vi "final-joystick.vi"() -> ()   [LabVIEW 2017]
uses:
  <vilib>/DAQmx/read.llb/DAQmx Read (Analog DBL 1Chan 1Samp).vi
  <vilib>/Utility/file.llb/Write Delimited Spreadsheet (string).vi
  <vilib>/Utility/file.llb/Read Delimited Spreadsheet (string).vi
  <vilib>/Utility/NIReport.llb/Append Report Text (str wrap).vi
  <vilib>/Utility/NIReport.llb/Append Text Table to Report (wrap).vi
  <vilib>/Utility/NIReport.llb/Append Image to Report (path wrap).vi
  <vilib>/DAQmx/create/channels.llb/DAQmx Create Channel (AI-Voltage-Basic).vi
  <vilib>/DAQmx/miscellaneous.llb/DAQmx Fill In Error Info.vi
  <vilib>/Utility/NIReport.llb/NI_report.lvclass
panel:
  in  "pos":string
  in  "x/y":string
  in  "File Path":path
  out "Array":string[][](array[string])
  out "Voltage Value":dbl(graph)
  out "Stop\nindicator":bool
  in  "LOG":bool
  out "Output Voltage":dbl format="%0.2f"
  in  "Stop Acquisition":bool
  in  "Input Channel":tag
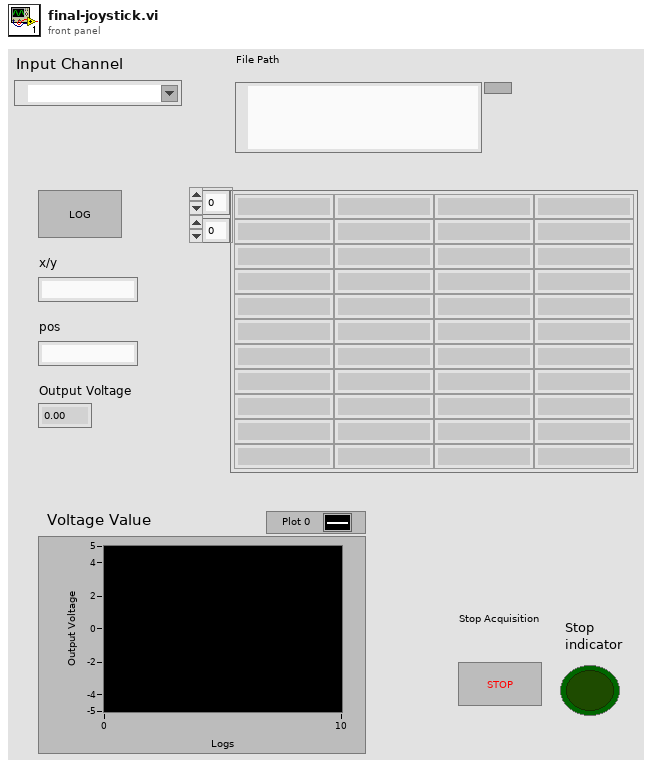
[diagram p1: front panel]
types:
  T1 = cluster{"Italic":enum16{"Italic Unchanged", "Italic On", "Italic Off"}, "Strike Through":enum16{"Strike Through Unchanged", "Strike Through On", "Strike Through Off"}, "Underline":enum16{"Underline Unchanged", "Underline On", "Underline Off"}, "Bold":enum16{"Bold Unchanged", "Bold On", "Bold Off"}}
  T2 = cluster{"Charset (-1)":i16, "Weight (-1)":i16, "Name":string, "Size":string}
  T3 = enum16{"maximized", "minimized", "normal", "no change"}
  T4 = enum16{"Standard Report", "HTML", "Word", "Excel"}
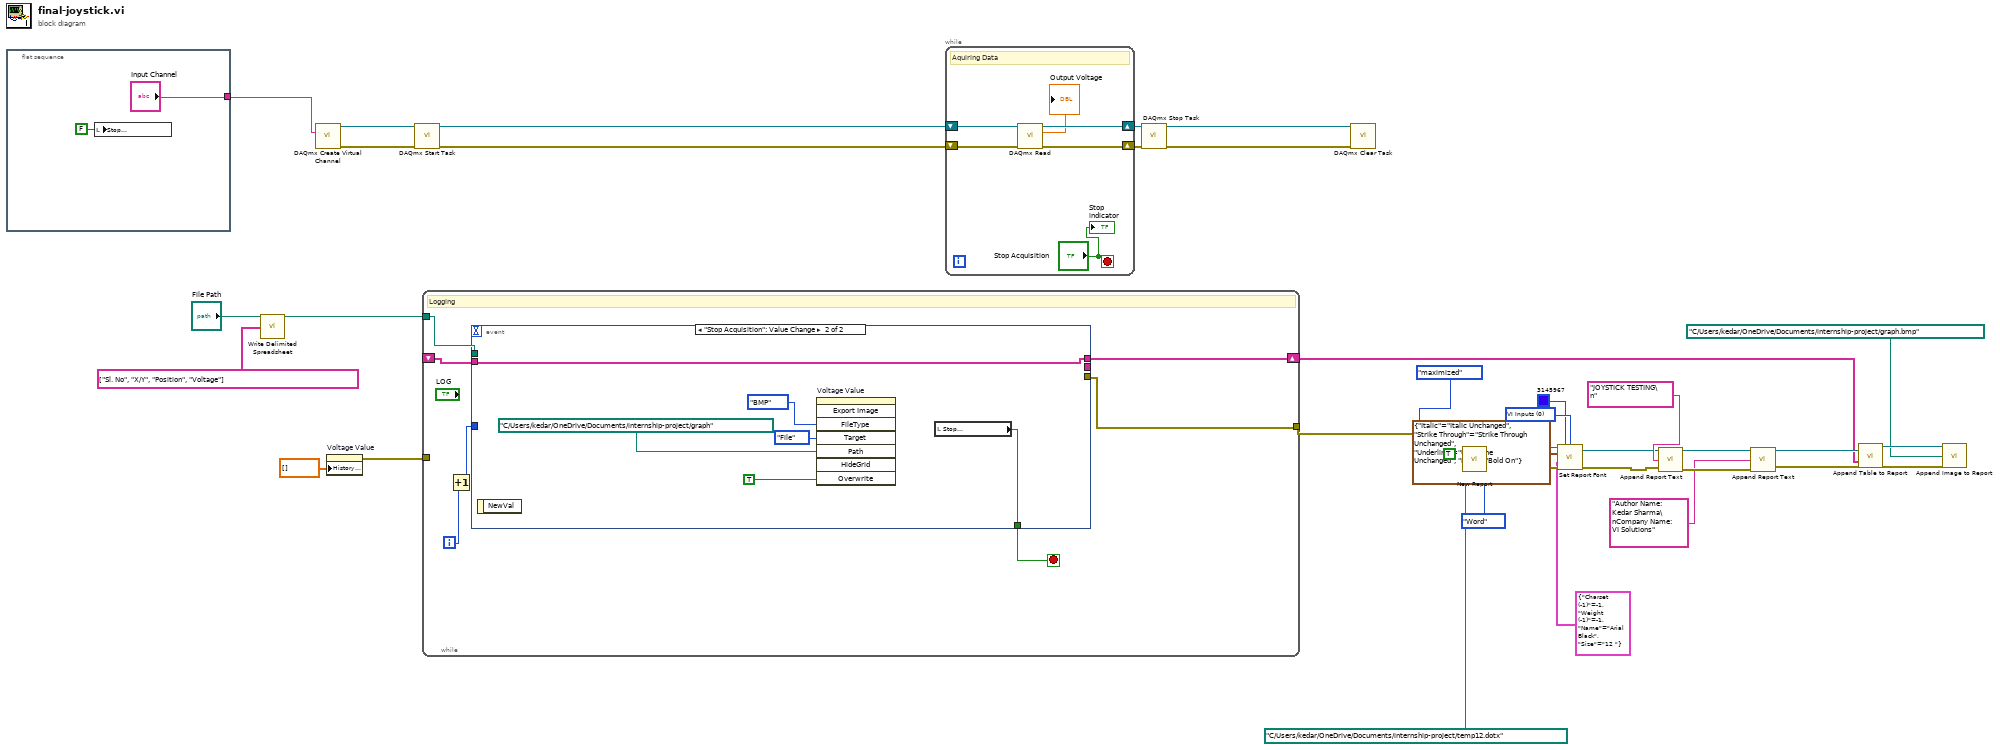
[diagram p0: block diagram]
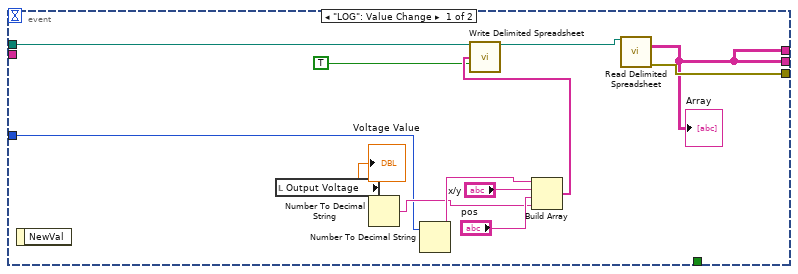
[diagram p2: hidden frame]
diagram:
  w2 = u16 0 items=["VI Inputs", "Font Dialog Box"] ("font settings source (VI Inputs)")
  n1 = flat-sequence {
    tunnel: ["Input Channel"] -> w29
    frame #0 {
      n2 = local write "Stop\nindicator"(FALSE ("Stop indicator")) -> ()
    }
  }
  n3 = call-poly <vilib>:"Write Delimited Spreadsheet.vi"("file path (dialog if empty)"="File Path", "1D data"=string[] ["Sl. No", "X/Y", "Position", "Voltage"]) -> ("new file path (Not A Path if cancelled)"=w25:path)  [unwired: 12 in, 1 out]
  n4 = call-poly <vilib>:"DAQmx Create Virtual Channel.vi"("physical channels"=w29) -> ("task out"=w37:refnum<k21>, "error out"=w36:errorcluster)  [unwired: 13 in]
  n5 = property on="Voltage Value" class="WFChart (strict)"("History Data"=dbl[] []) -> (error out=w27:errorcluster)  [unwired: 2 in, 1 out]
  n6 = call <vilib>:"DAQmx Start Task.vi"("task/channels in"=w37, "error in"=w36) -> ("task out"=w35:refnum<k21>, "error out"=w34:errorcluster)  [unwired: 12 in]
  n7 = while {
    tunnel: w27 -> [_]
    tunnel: w25 -> [w45]
    tunnel: [w42] -> w16
    shift-right: [w43] -> w15
    shift-left: _ -> [w40]
    i -> [w46]
    stop <- w41 stop-if-true
    # "Logging"
    n8 = Increment(x=w46) -> (x+1=w44:i32)
    n9 = event shown="[1] \"Stop Acquisition\": Value Change" {
      selector: _ -> [_ _]
      dyn-events: _ -> [_ _]
      timeout: _ -> [_ _]
      tunnel: w44 -> [w49 _]
      tunnel: w45 -> [w53 _]
      tunnel: [w47 _] -> _
      tunnel: [w48 _] -> w42
      tunnel: [w47 w59] -> w43
      tunnel: [_ w64] -> w41
      tunnel: w40 -> [_ w59]
      event "LOG": Value Change {
        n10 = event-data() -> ()  [unwired: 1 in, 1 out]
        n11 = local read "Output Voltage"() -> (w58:dbl)
        "Voltage Value" <- w58
        n12 = Number To Decimal String(number=w58) -> (decimal integer string=w54:string)  [unwired: 1 in]
        n13 = Number To Decimal String(number=w49) -> (decimal integer string=w56:string)  [unwired: 1 in]
        n14 = Build Array(w56, "x/y", "pos", w54) -> (w52:string[])
        n15 = call-poly <vilib>:"Write Delimited Spreadsheet.vi"("file path (dialog if empty)"=w53, "1D data"=w52, "append to file? (new file:F)"=TRUE) -> ("new file path (Not A Path if cancelled)"=w50:path)  [unwired: 11 in, 1 out]
        n16 = call-poly <vilib>:"Read Delimited Spreadsheet.vi"("file path (dialog if empty)"=w50) -> ("all rows"=w47:string[][], "error out"=w48:errorcluster)  [unwired: 9 in, 4 out]
        "Array" <- w47
      }
      event "Stop Acquisition": Value Change {
        n17 = event-data() -> ()  [unwired: 1 in, 1 out]
        n18 = invoke on="Voltage Value" class="WFChart (strict)" method="Export Image"("FileType"=enum32{"BMP", "EPS", "EMF", "PICT"}."BMP" ("File Type"), "Target"=enum32{"File", "Clipboard"}."File", "Path"=path "C:/Users/kedar/OneDrive/Documents/internship-project/graph", "Overwrite"=TRUE ("Always Overwrite")) -> ()  [unwired: 4 in, 8 out]
        n19 = local read "Stop\nindicator"() -> (w64:bool)
      }
    }
  }
  n20 = while {
    shift-right: [w68] -> w33
    shift-left: w35 -> [w70]
    shift-right: [w67] -> w32
    shift-left: w34 -> [w69]
    stop <- "Stop Acquisition" stop-if-true
    # "Aquiring Data"
    n21 = call-poly <vilib>:"DAQmx Read.vi"("task/channels in"=w70, "error in"=w69) -> ("task out"=w68:refnum<k21>, "data"=→"Output Voltage":dbl, "error out"=w67:errorcluster)  [unwired: 11 in]
    "Stop\nindicator" <- "Stop Acquisition"
  }
  n22 = call <vilib>:"DAQmx Stop Task.vi"("task/channels in"=w33, "error in"=w32) -> ("task out"=w31:refnum<k21>, "error out"=w30:errorcluster)  [unwired: 12 in]
  n23 = call <vilib>:"DAQmx Clear Task.vi"("task in"=w31, "error in"=w30) -> ()  [unwired: 13 in, 1 out]
  n24 = call <vilib>:"New Report.vi"("window state (normal)"=T3."maximized", "display alerts? (F)"=TRUE, "report type"=T4."Word", "template (empty)"=path "C:/Users/kedar/OneDrive/Documents/internship-project/temp12.dotx", "error in (no error)"=w16) -> ("report out"=w8:refnum<class "NI_report.lvclass">, "error out"=w6:errorcluster)  [unwired: 9 in]
  n25 = call-dynamic "Set Report Font.vi"("report in"=w8, "text color (unchanged)"=u32 3145967, "font settings source (VI Inputs)"=w2, "text options"=T1 {"Italic"=enum."Italic Unchanged", "Strike Through"=enum."Strike Through Unchanged", "Underline"=enum."Underline Unchanged", "Bold"=enum."Bold On"}, "font settings"=T2 {"Charset (-1)"=-1, "Weight (-1)"=-1, "Name"="Arial Black", "Size"="12 "}, "error in (no error)"=w6) -> ("report out"=w7:refnum<class "NI_report.lvclass">, "error out"=w5:errorcluster)  [unwired: 7 in, 1 out]
  n26 = call-poly <vilib>:"Append Report Text.vi"("report in"=w7, "text"="JOYSTICK TESTING\n" ("title"), "error in (no error)"=w5) -> ("report out"=w20:refnum<class "NI_report.lvclass">, "error out"=w21:errorcluster)  [unwired: 9 in, 2 out]
  n27 = call-poly <vilib>:"Append Report Text.vi"("report in"=w20, "text"="Author Name: Kedar Sharma\nCompany Name: VI Solutions", "error in (no error)"=w21) -> ("report out"=w22:refnum<class "NI_report.lvclass">, "error out"=w23:errorcluster)  [unwired: 9 in, 2 out]
  n28 = call-poly <vilib>:"Append Table to Report.vi"("report in"=w22, "text data"=w15, "error in (no error)"=w23) -> ("report out"=w13:refnum<class "NI_report.lvclass">, "error out"=w12:errorcluster)  [unwired: 9 in, 2 out]
  n29 = call-poly <vilib>:"Append Image to Report.vi"("report in"=w13, "path or URL of image"=path "C:/Users/kedar/OneDrive/Documents/internship-project/graph.bmp", "error in (no error)"=w12) -> ()  [unwired: 9 in, 4 out]
